vi "DCGlobals.vi"() -> ()   [LabVIEW 2020]
uses:
  <vilib>/variable/detnetvar/Network provider/DC2.llb/DCTerminalRefNum.ctl
  <vilib>/variable/detnetvar/Network provider/DC2.llb/DCDeviceRefNum.ctl
panel:
  in  "NodeId":string
  in  "Synchronization Progress":u8
  in  "Cycle Start TSrc Name":string
  in  "Device RefNum":T1 {"ID" format="%x"}
  in  "Terminal Ref Num":T2 {"ID" format="%x"}
  in  "Clock Sync Engine Error":errorcluster
  in  "Synced":bool
  out "Clock Sync vi reference":refnum<vi>
  in  "Log Engine Error":errorcluster
  out "Log Engine vi reference":refnum<vi>
  in  "Stop":bool
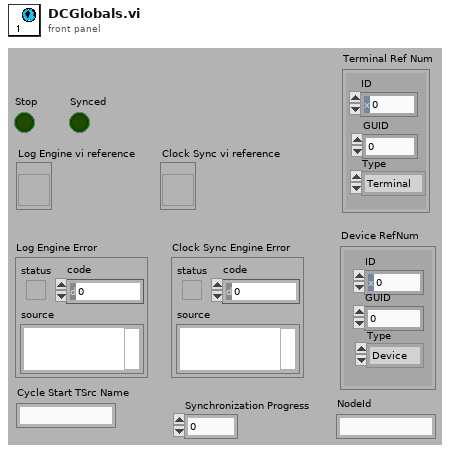
[diagram p1: front panel]
types:
  T1 = typedef "DCDeviceRefNum.ctl" = cluster{"ID":i32, "GUID":dbl, "Type":enum32{"Device"}}
  T2 = typedef "DCTerminalRefNum.ctl" = cluster{"ID":i32, "GUID":dbl, "Type":enum16{"Terminal"}}
diagram:
